vi "Copy .LLB to NI VeriStand dir.vi"(5 "Files Generated by Build":path[](array[path]), 6 "Top Level/Always Included VIs":path[](array[path]), 7 "Destination Path":path, 8 "error in (no error)":errorcluster, 9 "Target Name":string, 10 "Build Specification Name":string, 11 "Project Path":path) -> (0 "error out":errorcluster)   [LabVIEW 2024]
doc: "This VI is called after each run of a build specification. The VI will copy the generated LLB (Engine or System Explorer) into the VeriStand Custom Device folder (...\\Documents\\National Instruments\\NI VeriStand 2013...)."
uses:
  C:/Users/ppathak/Downloads/NationalInstruments.VeriStand.dll
  Users/ppathak/Downloads/NationalInstruments.VeriStand.dll
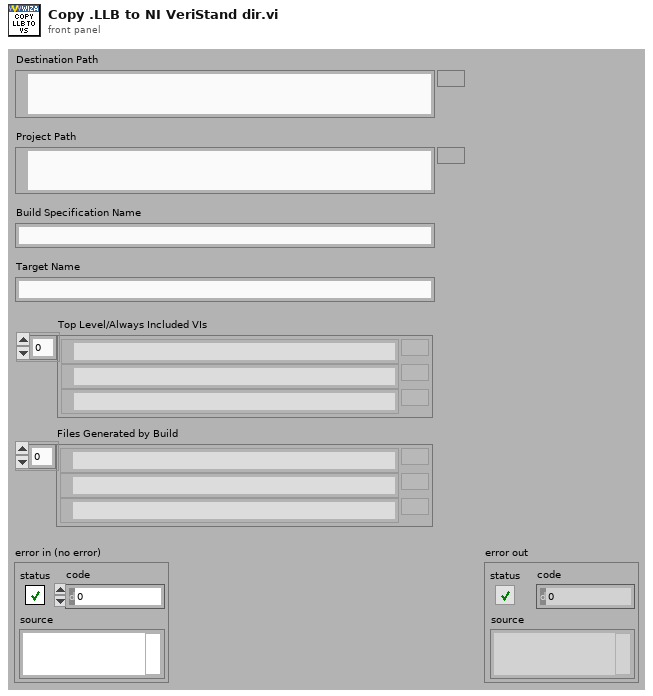
[diagram p1: front panel]
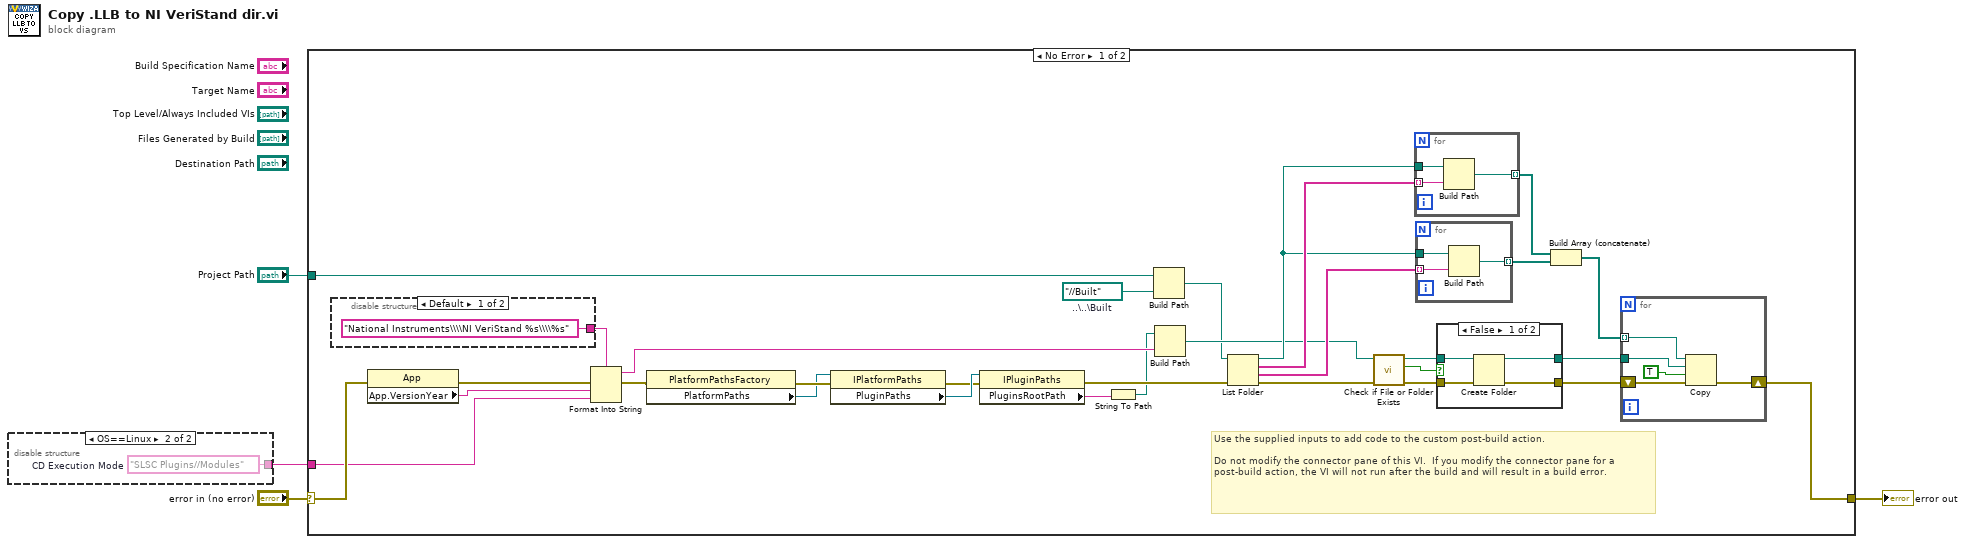
[diagram p0: block diagram]
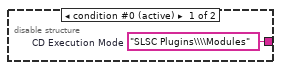
[diagram p2: hidden frame]
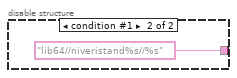
[diagram p3: hidden frame]
diagram:
  n1 = disable-structure shown="OS==Linux" {
    disable-tunnel: [w5 w6] -> w1
    frame condition #0 (active) {
      w5 = "SLSC Plugins\\\\Modules"  # CD Execution Mode
    }
    frame condition #1 {
      w6 = "SLSC Plugins//Modules"  # CD Execution Mode
    }
  }
  n2 = case shown="No Error" "error in (no error)" {
    selector: "error in (no error)" -> [w23 w57]
    tunnel: [w25 w57] -> w2
    tunnel: "Project Path" -> [w22 _]
    tunnel: w1 -> [w16 _]
    frame No Error {
      w15 = path "../../Built"  # ..\..\Built
      # "Use the supplied inputs to add code to the custom post-build action.\n\nDo not modify the connector pane of this VI.  If you modify the connector pane for a post-build action, the VI will not run after the build and will result in a build error."
      n3 = disable-structure shown="Default" {
        disable-tunnel: ["National Instruments\\\\NI VeriStand %s\\\\%s" ("name or relative path") "lib64//niveristand%s//%s" ("name or relative path")] -> w18
        frame condition #0 (active) {
        }
        frame condition #1 {
        }
      }
      n4 = property class="App"(error in=w23) -> (error out=w26:errorcluster, "App.VersionYear"=w17:string)  [unwired: 1 in, 1 out]
      n5 = Format Into String(format string=w18, error in=w26, w17, w16) -> (resulting string=w27:string, error out=w9:errorcluster)  [unwired: 1 in]
      n6 = property class="PlatformPathsFactory"(error in=w9) -> (error out=w12:errorcluster, "PlatformPaths"=w10:refnum<k24>)  [unwired: 1 in, 1 out]
      n7 = property class="IPlatformPaths"(reference=w10, error in=w12) -> (error out=w11:errorcluster, "PluginPaths"=w13:refnum<k24>)  [unwired: 1 out]
      n8 = property class="IPluginPaths"(reference=w13, error in=w11) -> (error out=w8:errorcluster, "PluginsRootPath"=w14:string)  [unwired: 1 out]
      n9 = String To Path(string=w14) -> (path=w7:path)
      n10 = Build Path(base path=w22, name or relative path=w15) -> (appended path=w19:path)
      n11 = Build Path(base path=w7, name or relative path=w27) -> (appended path=w24:path)
      n12 = List Folder(path=w19, error in=w8) -> (path out=w30:path, filenames=w37:string[], folder names=w31:string[], error out=w28:errorcluster)  [unwired: 2 in]
      n13 = call <vilib>:"Check if File or Folder Exists.vi"("error in (no error)"=w28, "path"=w24) -> ("error out"=w32:errorcluster, "file or folder exists?"=w34:bool, "dup path"=w33:path)  [unwired: 7 in]
      n14 = for {
        tunnel: w37 -> [w55] mode=indexing
        tunnel: w30 -> [w56]
        tunnel: [w54] -> w36 mode=indexing
        n15 = Build Path(base path=w56, name or relative path=w55) -> (appended path=w54:path)
      }
      n16 = for {
        tunnel: w31 -> [w52] mode=indexing
        tunnel: w30 -> [w53]
        tunnel: [w51] -> w29 mode=indexing
        n17 = Build Path(base path=w53, name or relative path=w52) -> (appended path=w51:path)
      }
      n18 = case shown="False" w34 {
        tunnel: w33 -> [w43 w45]
        tunnel: w32 -> [w42 w44]
        tunnel: [w41 w45] -> w21
        tunnel: [w40 w44] -> w20
        frame False {
          n19 = Create Folder(path (use dialog)=w43, error in=w42) -> (created path=w41:path, error out=w40:errorcluster)  [unwired: 1 in, 1 out]
        }
        frame True {
        }
      }
      n20 = Build Array (concatenate)(w36, w29) -> (w35:path[])
      n21 = for {
        tunnel: w35 -> [w47] mode=indexing
        shift-right: [w48] -> w25
        shift-left: w20 -> [w49]
        tunnel: w21 -> [w46]
        n22 = Copy(8:w49, 9:TRUE ("overwrite (F)"), 10:w46, 11:w47) -> (0:w48:errorcluster)  [unwired: 1 in, 2 out]
      }
    }
    frame Error {
    }
  }
  "error out" <- w2
